vi "create_files.vi"(0 "base path":path, 1 "cell number string":string) -> (2 "dc resistance log file path":path, 3 "raw data log file path":path, 4 "charge state log file path":path, 5 "discharge state log file path":path, 6 "predischarge state log file path":path, 7 "postcharge state log file path":path)   [LabVIEW 2016]
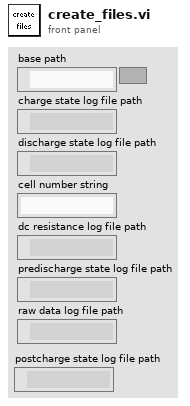
[diagram p1: front panel]
types:
  T1 = enum16{"open", "open or create", "create or replace", "create", "open (read only)"}
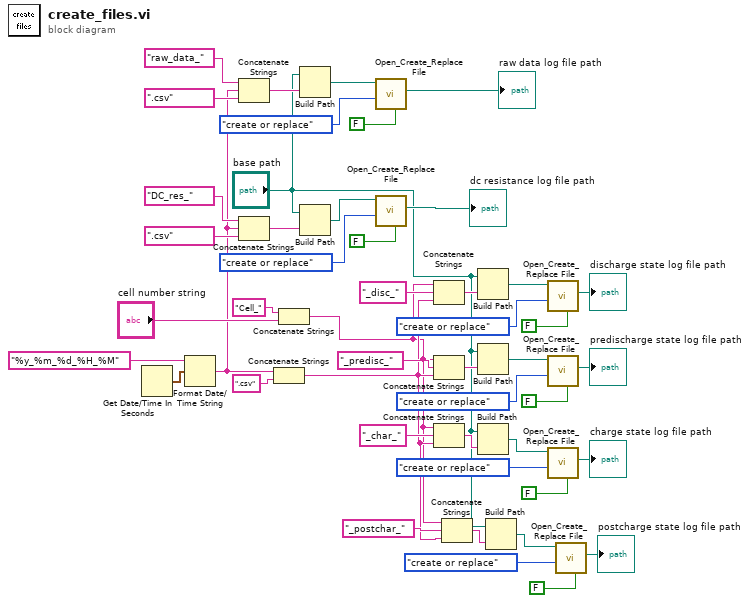
[diagram p0: block diagram]
diagram:
  n1 = Get Date/Time In Seconds() -> (seconds since 1Jan1904=w32:timestamp)
  n2 = Format Date/Time String(time format string (%c)="%y_%m_%d_%H_%M", seconds (now)=w32) -> (date/time string=w12:string)  [unwired: 1 in]
  n3 = Concatenate Strings("raw_data_", w12, ".csv") -> (w18:string)
  n4 = Concatenate Strings("DC_res_", w12, ".csv") -> (w24:string)
  n5 = Concatenate Strings(w12, ".csv" ("string")) -> (w3:string)
  n6 = Concatenate Strings("Cell_" ("string"), "cell number string") -> (w2:string)
  n7 = Build Path(base path="base path", name or relative path=w18) -> (appended path=w15:path)
  n8 = Build Path(base path="base path", name or relative path=w24) -> (appended path=w21:path)
  n9 = call <vilib>:"Open_Create_Replace File.vi"("advisory dialog? (display:T)"=FALSE, "function (open:0)"=T1."create or replace", "file path"=w15) -> ("new file path"=→"raw data log file path":path)  [unwired: 5 in, 3 out]
  n10 = call <vilib>:"Open_Create_Replace File.vi"("advisory dialog? (display:T)"=FALSE, "function (open:0)"=T1."create or replace", "file path"=w21) -> ("new file path"=→"dc resistance log file path":path)  [unwired: 5 in, 3 out]
  n11 = Concatenate Strings(w2, "_disc_", w3) -> (w45:string)
  n12 = Concatenate Strings(w2, "_predisc_", w3) -> (w44:string)
  n13 = Concatenate Strings(w2, "_char_", w3) -> (w46:string)
  n14 = Concatenate Strings(w2, "_postchar_", w3) -> (w9:string)
  n15 = Build Path(base path="base path", name or relative path=w45) -> (appended path=w30:path)
  n16 = Build Path(base path="base path", name or relative path=w44) -> (appended path=w37:path)
  n17 = Build Path(base path="base path", name or relative path=w46) -> (appended path=w31:path)
  n18 = Build Path(base path="base path", name or relative path=w9) -> (appended path=w7:path)
  n19 = call <vilib>:"Open_Create_Replace File.vi"("advisory dialog? (display:T)"=FALSE, "function (open:0)"=T1."create or replace", "file path"=w30) -> ("new file path"=→"discharge state log file path":path)  [unwired: 5 in, 3 out]
  n20 = call <vilib>:"Open_Create_Replace File.vi"("advisory dialog? (display:T)"=FALSE, "function (open:0)"=T1."create or replace", "file path"=w37) -> ("new file path"=→"predischarge state log file path":path)  [unwired: 5 in, 3 out]
  n21 = call <vilib>:"Open_Create_Replace File.vi"("advisory dialog? (display:T)"=FALSE, "function (open:0)"=T1."create or replace", "file path"=w31) -> ("new file path"=→"charge state log file path":path)  [unwired: 5 in, 3 out]
  n22 = call <vilib>:"Open_Create_Replace File.vi"("advisory dialog? (display:T)"=FALSE, "function (open:0)"=T1."create or replace", "file path"=w7) -> ("new file path"=→"postcharge state log file path":path)  [unwired: 5 in, 3 out]
